vi "Queue Comms Dequeue.vi"(8 "error in":errorcluster) -> (0 "error out":errorcluster, 3 "element":T1)   [LabVIEW 2018, in "Error Handler.lvlib"]
doc: "This subVI dequeues an element from the communications queue using the Queue Comms FGV"
uses:
  Error Handler.lvlib
  Private Controls/Module Data.ctl
  Private Controls/Module Action.ctl
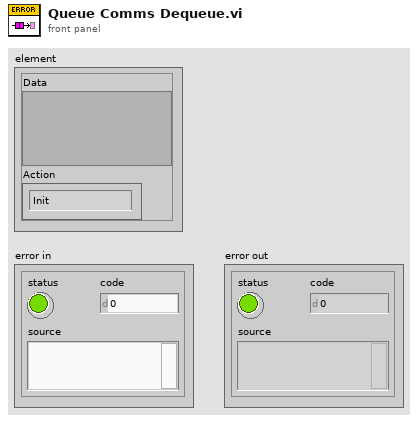
[diagram p1: front panel]
types:
  T1 = typedef "Error Handler.lvlib/Module Data.ctl" = cluster{"Data":variant, "Action":T2}
  T2 = typedef "Error Handler.lvlib/Module Action.ctl" = enum8{"Init", "Exit", "Controller Error", "UI1 Error", "UI2 Error", "UI3 Error", "File IO Error", "cRIO Error", "Calibration Error"}
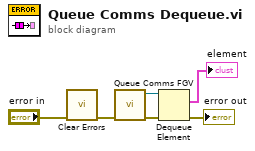
[diagram p0: block diagram]
diagram:
  n1 = call <vilib>:"Clear Errors.vi"("error in (no error)"="error in") -> ("error out"=w1:errorcluster)  [unwired: 5 in, 1 out]
  n2 = call "Queue Comms FGV.vi"("error in (no error)"=w1) -> ("error out"=w6:errorcluster, "Queue out"=w5:refnum<queue>)  [unwired: 9 in]
  n3 = Dequeue Element(queue=w5, error in (no error)=w6) -> (element=→"element":T1, error out=→"error out":errorcluster)  [unwired: 1 in, 2 out]
